vi "Configure TV Trigger Source.vi"(0 "VISA Resource Name":refnum<visa-resource-name>, 5 "Trigger Source (Channel 1)":string(combo)="CH1", 7 "TV Trigger Signal Format (NTSC)":i32(slide), 9 "TV Event (Field 1)":i32(slide), 11 "error in (no error)":errorcluster {"code" format="%.0x"}) -> (4 "VISA Resource Name Out":refnum<visa-resource-name>, 15 "error out":errorcluster {"code" format="%.0x"})   [LabVIEW 2010, in "Tektronix TDS 3000 Series.lvlib"]
doc: "This VI configures the TV trigger. You configure the TV trigger source, signal format, the event on which to trigger, and the signal polarity.\n\nNotes:\n\n(1) This VI affects instrument behavior only if the Trigger Type is TV Trigger. Call the Configure Trigger VI to set the Trigger Type before you call this VI."
uses:
  <instrlib>/Tektronix TDS 3000 Series/Tektronix TDS 3000 Series.lvlib
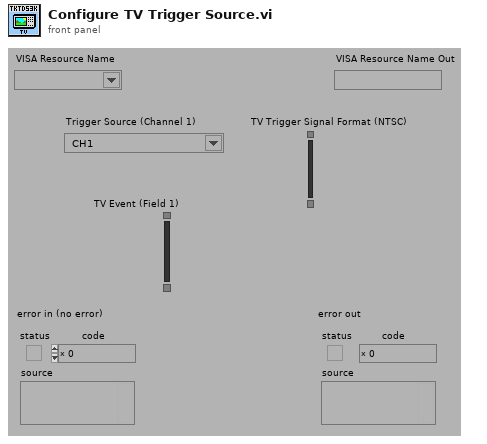
[diagram p1: front panel]
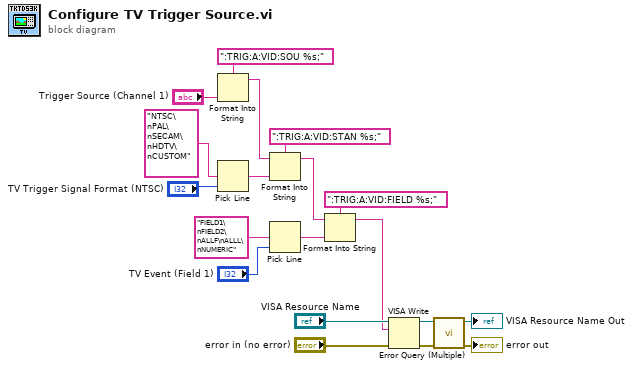
[diagram p0: block diagram]
diagram:
  n1 = Format Into String(format string=":TRIG:A:VID:SOU %s;", "Trigger Source (Channel 1)") -> (resulting string=w11:string)  [unwired: 2 in, 1 out]
  n2 = Pick Line(multi-line string="NTSC\nPAL\nSECAM\nHDTV\nCUSTOM", line index="TV Trigger Signal Format (NTSC)") -> (output string=w12:string)  [unwired: 1 in]
  n3 = Format Into String(format string=":TRIG:A:VID:STAN %s;", initial string=w11, w12) -> (resulting string=w7:string)  [unwired: 1 in, 1 out]
  n4 = Pick Line(multi-line string="FIELD1\nFIELD2\nALLF\nALLL\nNUMERIC", line index="TV Event (Field 1)") -> (output string=w8:string)  [unwired: 1 in]
  n5 = Format Into String(format string=":TRIG:A:VID:FIELD %s;", initial string=w7, w8) -> (resulting string=w6:string)  [unwired: 1 in, 1 out]
  n6 = VISA Write(VISA resource name="VISA Resource Name", write buffer=w6, error in (no error)="error in (no error)") -> (VISA resource name out=w4:refnum<visa-resource-name>, error out=w3:errorcluster)  [unwired: 1 out]
  n7 = call <instrlib>:"Error Query (Multiple).vi"("error in (no error)"=w3, "VISA Resource Name"=w4) -> ("error out"=→"error out":errorcluster, "VISA Resource Name Out"=→"VISA Resource Name Out":refnum<visa-resource-name>)  [unwired: 6 in, 2 out]
